vi "Datalogging.vi"   [LabVIEW 2019]
uses:
  <vilib>/Rock Robotics/WPI/ThirdParty/Phoenix-LabVIEW/Motor Controller/Get/CTRE_Phoenix_MotorController_GetSelectedSensorData.vi
  Infinite Recharge current/Robot Global Data.vi
  <vilib>/Utility/file.llb/Write Delimited Spreadsheet (string).vi
types:
  T1 = typedef "WPI_MotorControlDeviceRef.ctl" = cluster{"DeviceStatus":errorcluster, "Type":T2, "PWM":cluster{"PWM Channel":T3, "DeadBand":T4}, "CAN":cluster{"Device Number":u8, "SetOutput VI Ref":variant, "GetOutput VI Ref":variant, "Enable VI Ref":variant, "Disable VI Ref":variant, "Data":variant}, "Invert":bool, "DIO PWM":cluster{"PWM \"Enable\" Channel":T3, "DIOChannel":T5, "PWM Rate":dbl}}
  T2 = typedef "WPI_MotorControlType.ctl" = enum16{"PWM", "CAN", "DIO PWM"}
  T3 = typedef "FPGA_DIOPWMChannel.ctl" = enum8{"PWM 0", "PWM 1", "PWM 2", "PWM 3", "PWM 4", "PWM 5", "PWM 6", "PWM 7", "PWM 8", "PWM 9", "PWM MXP 0", "PWM MXP 1", "PWM MXP 2", "PWM MXP 3", "PWM MXP 4", "PWM MXP 5", "PWM MXP 6", "PWM MXP 7", "PWM MXP 8", "PWM MXP 9", "Invalid"}
  T4 = typedef "WPI_PWMDeadband.ctl" = cluster{"Name":string, "maxPositivePwm":i32, "minPositivePwm":i32, "centerPwm":i32, "maxNegativePwm":i32, "minNegativePwm":i32, "angularRange":u16}
  T5 = typedef "FPGA_DIOChannel.ctl" = enum8{"DIO 0", "DIO 1", "DIO 2", "DIO 3", "DIO 4", "DIO 5", "DIO 6", "DIO 7", "DIO 8", "DIO 9", "DIO MXP 0", "DIO MXP 1", "DIO MXP 2", "DIO MXP 3", "DIO MXP 4", "DIO MXP 5", "DIO MXP 6", "DIO MXP 7", "DIO MXP 8", "DIO MXP 9", "DIO MXP 10", "DIO MXP 11", "DIO MXP 12", "DIO MXP 13", "DIO MXP 14", "DIO MXP 15", "SPI Port CS1", "SPI Port CS2", "SPI Port CS3", "SPI Port MISO", "SPI Port MOSI", "Invalid"}
  T6 = cluster{"Yaw":dbl, "Roll":dbl, "Pitch":dbl, "Heading":dbl, "Fused Heading":dbl}
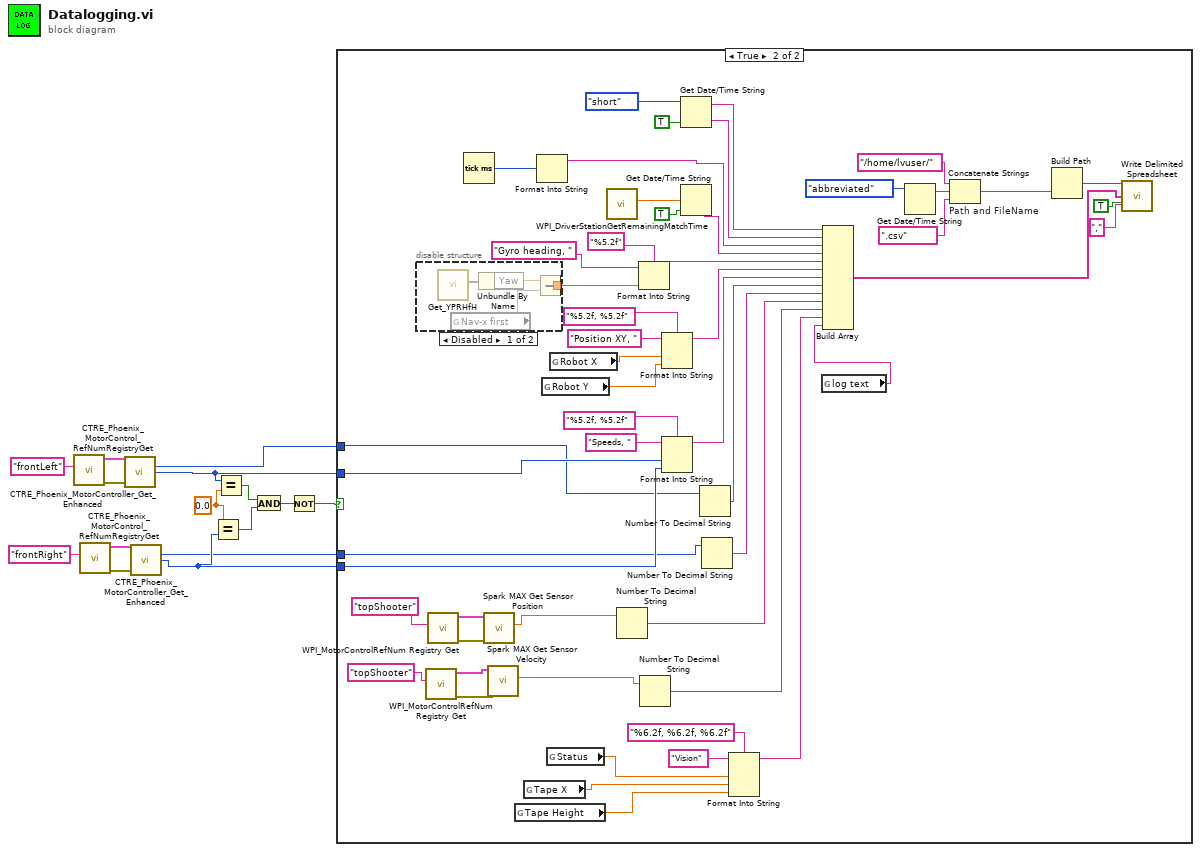
[diagram p0: block diagram]
diagram:
  w15 = 0.0 ("y")
  n1 = call <vilib>:"CTRE_Phoenix_MotorControl_RefNumRegistryGet.vi"("refnum name"="frontLeft") -> ("error out"=w10:errorcluster, "PhoenixMotorControlDevRef"=w9:T1)  [unwired: 9 in]
  n2 = call <vilib>:"CTRE_Phoenix_MotorControl_RefNumRegistryGet.vi"("refnum name"="frontRight") -> ("error out"=w6:errorcluster, "PhoenixMotorControlDevRef"=w5:T1)  [unwired: 9 in]
  n3 = call-poly <vilib>:"CTRE_Phoenix_MotorController_Get_Enhanced.vi"("PhoenixMotorControlDevRef"=w9, "error in"=w10) -> ("Position (Raw Sensor Units)"=w2:i32, "Velocity (Raw Sensor Units per 100 ms)"=w7:i32)  [unwired: 10 in, 2 out]
  n4 = call-poly <vilib>:"CTRE_Phoenix_MotorController_Get_Enhanced.vi"("PhoenixMotorControlDevRef"=w5, "error in"=w6) -> ("Position (Raw Sensor Units)"=w1:i32, "Velocity (Raw Sensor Units per 100 ms)"=w3:i32)  [unwired: 10 in, 2 out]
  n5 = Equal?(x=w15, y=w3) -> (x = y?=w13:bool)
  n6 = Equal?(x=w7, y=w15) -> (x = y?=w14:bool)
  n7 = And(x=w14, y=w13) -> (x .and. y?=w12:bool)
  n8 = Not(x=w12) -> (.not. x?=w11:bool)
  n9 = case shown="True" w11 {
    tunnel: w7 -> [_ w41]
    tunnel: w3 -> [_ w40]
    tunnel: w2 -> [_ w39]
    tunnel: w1 -> [_ w38]
    frame False {
    }
    frame True {
      n10 = disable-structure shown="Disabled" {
        disable-tunnel: [w69 _] -> w62
        frame Disabled {
          n11 = call <vilib>:"Get_YPRHfH.vi"() -> ("YRPHfH"=w70:T6)  [unwired: 11 in]
          n12 = global read "Robot Global Data.vi" "Nav-x first"() -> (w72)
          n13 = Unbundle By Name(w70) -> ("Yaw"=w71:dbl)
          n14 = Subtract(x=w71, y=w72) -> (x-y=w69:dbl)
        }
        frame Enabled {
        }
      }
      n15 = call <vilib>:"WPI_MotorControlRefNum Registry Get.vi"("refnum name"="topShooter") -> ("error out"=w27:errorcluster, "MotorControlDevRef"=w28:T1)  [unwired: 9 in]
      n16 = call <vilib>:"WPI_MotorControlRefNum Registry Get.vi"("refnum name"="topShooter") -> ("error out"=w30:errorcluster, "MotorControlDevRef"=w29:T1)  [unwired: 9 in]
      n17 = Tick Count (ms)() -> (millisecond timer value=w43:u32)
      n18 = call <vilib>:"Spark MAX Get Sensor Position.vi"("error in (no error)"=w30, "MotorControlDevRef in"=w29) -> ("Sensor Position"=w17:dbl)  [unwired: 6 in, 3 out]
      n19 = call <vilib>:"Spark MAX Get Sensor Velocity.vi"("error in (no error)"=w27, "MotorControlDevRef in"=w28) -> ("Sensor Velocity"=w16:dbl)  [unwired: 6 in, 3 out]
      n20 = global read "Robot Global Data.vi" "Tape Height"() -> (w22:dbl)
      n21 = global read "Robot Global Data.vi" "Tape X"() -> (w21:dbl)
      n22 = Format Into String(w43) -> (resulting string=w42:string)  [unwired: 3 in, 1 out]
      n23 = global read "Robot Global Data.vi" "Robot Y"() -> (w19:dbl)
      n24 = global read "Robot Global Data.vi" "Status"() -> (w23:dbl)
      n25 = global read "Robot Global Data.vi" "Robot X"() -> (w20:dbl)
      n26 = call <vilib>:"WPI_DriverStationGetRemainingMatchTime.vi"() -> ("Match Time(s)"=w68:sgl)  [unwired: 10 in, 1 out]
      n27 = Number To Decimal String(number=w17) -> (decimal integer string=w35:string)  [unwired: 1 in]
      n28 = Format Into String(format string="%5.2f", initial string="Gyro heading, " ("element"), w62) -> (resulting string=w46:string)  [unwired: 1 in, 1 out]
      n29 = Number To Decimal String(number=w16) -> (decimal integer string=w34:string)  [unwired: 1 in]
      n30 = Format Into String(format string="%5.2f, %5.2f", initial string="Position XY, ", w20, w19) -> (resulting string=w45:string)  [unwired: 1 in, 1 out]
      n31 = Format Into String(format string="%5.2f, %5.2f", initial string="Speeds, ", w41, w40) -> (resulting string=w44:string)  [unwired: 1 in, 1 out]
      n32 = Get Date/Time String(date format (0)=enum16{"short", "long", "abbreviated"}."short", want seconds? (F)=TRUE) -> (date string=w55:string, time string=w54:string)  [unwired: 1 in]
      n33 = Get Date/Time String(seconds (now)=w68, want seconds? (F)=TRUE) -> (time string=w64:string)  [unwired: 1 in, 1 out]
      n34 = Number To Decimal String(number=w39) -> (decimal integer string=w37:string)  [unwired: 1 in]
      n35 = Number To Decimal String(number=w38) -> (decimal integer string=w36:string)  [unwired: 1 in]
      n36 = Format Into String(format string="%6.2f, %6.2f, %6.2f", initial string="Vision", w23, w21, w22) -> (resulting string=w31:string)  [unwired: 1 in, 1 out]
      n37 = global read "Robot Global Data.vi" "log text"() -> (w18:string)
      n38 = Build Array(w55, w54, w42, w64, w46, w45, w44, w37, w36, w35, w34, w31, w18) -> (w24:string[])
      n39 = Get Date/Time String(date format (0)=enum16{"short", "long", "abbreviated"}."abbreviated") -> (date string=w56:string)  [unwired: 2 in, 1 out]
      n40 = Concatenate Strings "Path and FileName"("/home/lvuser/", w56, ".csv") -> (w59:string)
      n41 = Build Path(name or relative path=w59) -> (appended path=w58:path)  [unwired: 1 in]
      n42 = call-poly <vilib>:"Write Delimited Spreadsheet.vi"("file path (dialog if empty)"=w58, "1D data"=w24, "append to file? (new file:F)"=TRUE, "delimiter (\\t)"="," ("delimiter (\\t)")) -> ()  [unwired: 10 in, 2 out]
    }
  }
